vi "Connect.vi"(6 "RC Type":T1, 8 "error in (no error)":errorcluster, 9 "Port":u16, 10 "address":string, 11 "RemoteControl in":refnum<class "RemoteControl.lvclass">) -> (0 "error out":errorcluster, 3 "RemoteControl out":refnum<class "RemoteControl.lvclass">)   [LabVIEW 2019, in "RemoteControl.lvclass"]
uses:
  RemoteControl.lvclass
  Typedefs/RC Com Type--enum.ctl
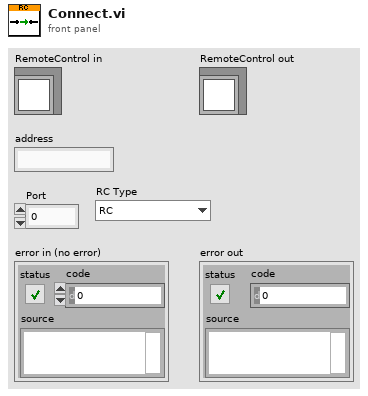
[diagram p1: front panel]
types:
  T1 = typedef "RemoteControl.lvclass/RC Com Type--enum.ctl" = enum16{"RC", "STM", "ZMQ"}
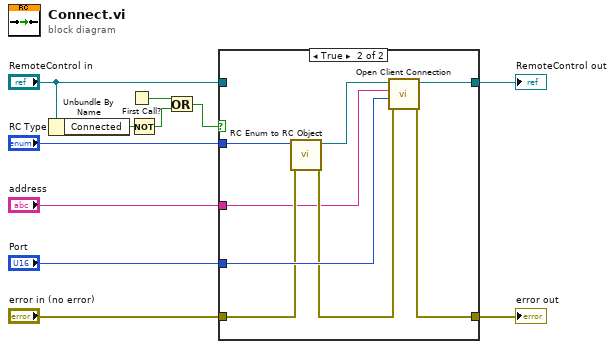
[diagram p0: block diagram]
diagram:
  n1 = Unbundle By Name("RemoteControl in") -> ("Connected"=w2:bool)
  n2 = First Call?() -> (First Call?: T/F=w4:bool)
  n3 = Not(x=w2) -> (.not. x?=w1:bool)
  n4 = Or(x=w4, y=w1) -> (x .or. y?=w3:bool)
  n5 = case shown="True" w3 {
    tunnel: [w12 w21] -> w11
    tunnel: "error in (no error)" -> [w12 w16]
    tunnel: [w13 w20] -> w9
    tunnel: "address" -> [_ w14]
    tunnel: "Port" -> [_ w19]
    tunnel: "RC Type" -> [_ w18]
    tunnel: "RemoteControl in" -> [w13 _]
    frame False {
    }
    frame True {
      n6 = call "RC Enum to RC Object.vi"("error in (no error)"=w16, "RC Type"=w18) -> ("error out"=w15:errorcluster, "RemoteControl out"=w17:refnum<class "RemoteControl.lvclass">)  [unwired: 8 in]
      n7 = call-dynamic "Open Client Connection.vi"("error in (no error)"=w15, "Port"=w19, "address"=w14, "RemoteControl in"=w17) -> ("error out"=w21:errorcluster, "RemoteControl out"=w20:refnum<class "RemoteControl.lvclass">)  [unwired: 6 in]
    }
  }
  "error out" <- w11
  "RemoteControl out" <- w9
